vi "Destroy.vi"(0 "reference":refnum<class "NoteNode.lvclass">, 5 "error in (no error)":errorcluster) -> (15 "# of objects":i32, 19 "error out":errorcluster)   [LabVIEW 2014, in "NoteNode.lvclass"]
doc: "Destroys a NoteNode object created with a NoteNode constructor VI.\n\n[GOOP 2.1]"
uses:
  <resource>/Framework/Providers/Open_GDS/UML/NoteNode_class/NoteNode.lvclass
  <resource>/Framework/Providers/Open_GDS/UML/RectangularNode_class/RectangularNode.lvclass
  <resource>/Framework/Providers/Open_GDS/UML/MultiLineString_class/MultiLineString.lvclass
panel:
  out "reference out":refnum<class "NoteNode.lvclass">
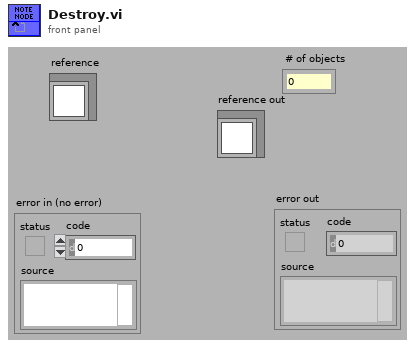
[diagram p1: front panel]
types:
  T1 = typedef "NoteNode.lvclass/ObjectAttributes.ctl" = cluster{"Base class":T2, "DEFAULT_WIDTH":i32, "DEFAULT_HEIGHT":i32, "DEFAULT_COLOR":u32, "FOLD_X":i32, "FOLD_Y":i32, "color":u32, "text":refnum<class "MultiLineString.lvclass">, "pointNodes":refnum<class "AbstractNode.lvclass">[]}
  T2 = typedef "RectangularNode.lvclass/ObjectAttributes.ctl" = cluster{"Base class":T3, "bounds":T4}
  T3 = typedef "AbstractNode.lvclass/ObjectAttributes.ctl" = cluster{"parent":refnum<class "AbstractNode.lvclass">, "children":refnum<class "AbstractNode.lvclass">[], "Hidden":bool}
  T4 = typedef "Rectangle Rectangle2D.ctl" = cluster{"x":dbl, "y":dbl, "width":dbl, "height":dbl}
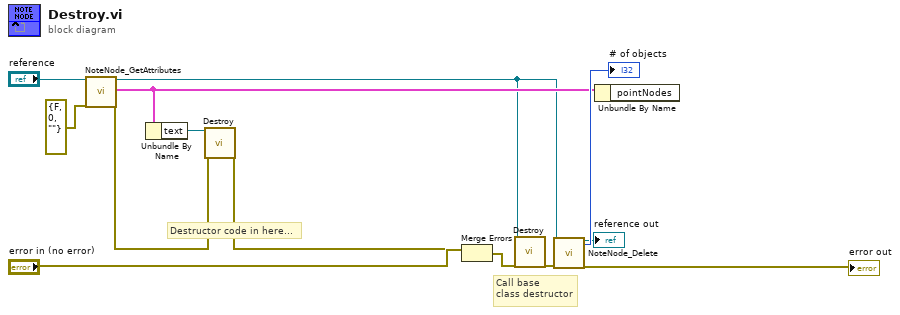
[diagram p0: block diagram]
diagram:
  # "Call base\nclass destructor"
  # "Destructor code in here..."
  n1 = call <resource>:"NoteNode_GetAttributes.vi"("reference in"="reference", "error in (no error)"=errorcluster {"status"=FALSE, "code"=0, "source"=""}) -> ("reference out"=w1:refnum<class "NoteNode.lvclass">, "Attributes"=w6:T1, "error out"=w8:errorcluster)  [unwired: 15 out]
  n2 = Unbundle By Name(w6) -> ("text"=w9:refnum<class "MultiLineString.lvclass">)
  n3 = call-dynamic "Destroy.vi"("reference"=w9, "error in (no error)"=w8) -> ("error out"=w7:errorcluster)  [unwired: 16 in, 1 out]
  n4 = Merge Errors("error in (no error)", w7) -> (w2:errorcluster)
  n5 = call-parent "Destroy.vi"("reference"=w1, "error in (no error)"=w2) -> ("error out"=w3:errorcluster)  [unwired: 16 in, 1 out]
  n6 = call <resource>:"NoteNode_Delete.vi"("reference in"=w1, "error in (no error)"=w3) -> ("reference out"=→"reference out":refnum<class "NoteNode.lvclass">, "# of objects"=→"# of objects":i32, "error out"=→"error out":errorcluster)  [unwired: 15 out]
  n7 = Unbundle By Name(w6) -> ()  [unwired: 1 out]
